vi "ChiSquareCalculation Uncalibrated Method.vi"(9 "refractive index, imaginary":dbl=0.037 format="%.5f", 10 "refractive index, real":dbl=1.567 format="%.5f", 11 "Extinction ExtinctionUncertainity Size parameter and Number ofS sizes 2":T2={"Extinction"=[1.8535327e-09, 2.3370865e-09, 2.8756633e-09, 3.369798e-09, 3.9789465e-09], "Extinction Uncertainty"=[2.1120453e-11, 4.1097261e-11, 5.5818728e-11, 7.3813344e-11, 9.5925372e-11], "Size parameters"=[2.3425015041273096, 2.5554561863207015, 2.7684108685140933, 2.9813655507074848, 3.194320232900877], "Number ofSizes"=5.0, "GeometricCrossSection"=[5.939573610693203e-10, 7.068583470577035e-10, 8.295768100885549e-10, 9.621127501618742e-10, 1.1044661672776617e-09], "Wave Length"=368.81, "SMPS Sizes"=[105.5, 109.4, 113.4, 117.6, 121.9, 126.3, 131.0, 135.8, 140.7, 145.9, 151.2, 156.8, 162.5, 168.5, 174.7, 181.1, 187.7, 194.6, 201.7, 209.1, 216.7, 224.7, 232.9, 241.4, 250.3, 259.5, 269.0, 278.8, 289.0, 299.6, 310.6, 322.0, 333.8, 346.0, 358.7, 371.8, 385.4, 399.5, 414.2, 429.4, 445.1, 461.4, 478.3, 495.8, 514.0, 532.8, 552.3, 572.5, 593.5, 615.3, 637.8, 661.2, 685.4, 710.5, 736.5, 763.5, 791.5], "Concentration"=[[0.0, 0.0, 0.0, 0.0, 0.0, 0.0, 0.0, 0.0, 0.0, 0.0, 0.0, 0.0, 0.0, 0.0, 0.0, 0.0, 0.0, 0.0, 0.0, 0.0, 0.0, 0.0, 0.0, 0.00638904, 0.0448604, 0.138777, 0.238948, 0.258203, 0.179447, 0.0783806, 0.0207428, 0.00279106, 0.000128936, 0.0, 0.0, 0.0, 0.0, 0.00019549, 0.00132468, 0.00397525, 0.00699496, 0.00773861, 0.00587311, 0.00303416, 0.00102868, 0.000183263, 2.21568e-05, 5.32123e-05, 0.000149497, 0.000216876, 0.00023158, 0.000165064, 9.50711e-05, 3.99013e-05, 8.12868e-06, 1.38253e-06, 1.50421e-07], [0.0, 0.0, 0.0, 0.0, 0.0, 0.0, 0.0, 0.0, 0.0, 0.0, 0.0, 0.0, 0.0, 0.0, 0.0, 0.0, 0.0, 0.0, 0.0, 0.0, 0.0, 0.0, 0.0, 0.0, 0.0, 0.00685673, 0.0470895, 0.141594, 0.242879, 0.258016, 0.178865, 0.0777681, 0.0205487, 0.00285525, 0.000153554, 0.0, 0.0, 0.0, 0.0, 0.000111464, 0.00081094, 0.00255922, 0.00482553, 0.00593792, 0.00495016, 0.00247994, 0.000820378, 0.000203601, 2.54423e-05, 1.65921e-05, 5.51241e-05, 0.000106166, 0.000152004, 0.000157397, 8.55848e-05, 5.09931e-05, 2.62187e-05], [0.0, 0.0, 0.0, 0.0, 0.0, 0.0, 0.0, 0.0, 0.0, 0.0, 0.0, 0.0, 0.0, 0.0, 0.0, 0.0, 0.0, 0.0, 0.0, 0.0, 0.0, 0.0, 0.0, 0.0, 0.0, 0.0, 0.0, 0.0072478, 0.0494094, 0.145408, 0.247245, 0.258864, 0.175884, 0.0757159, 0.0204247, 0.00297997, 0.000182238, 0.0, 0.0, 0.0, 0.0, 4.50403e-05, 0.000404956, 0.00155479, 0.00339027, 0.0041382, 0.00335173, 0.00222974, 0.000866046, 0.000189774, 2.77835e-05, 5.5897e-06, 2.322e-05, 6.96631e-05, 9.61216e-05, 0.000135395, 0.000110007], [0.0, 0.0, 0.0, 0.0, 0.0, 0.0, 0.0, 0.0, 0.0, 0.0, 0.0, 0.0, 0.0, 0.0, 0.0, 0.0, 0.0, 0.0, 0.0, 0.0, 0.0, 0.0, 0.0, 0.0, 0.0, 0.0, 0.0, 0.0, 0.0, 0.00780939, 0.0525691, 0.151633, 0.250554, 0.256059, 0.173088, 0.0742833, 0.0201712, 0.00304534, 0.000198007, 0.0, 0.0, 0.0, 0.0, 0.0, 0.000142408, 0.000753018, 0.00176172, 0.00291712, 0.00270485, 0.00146477, 0.000603494, 0.000160512, 3.03021e-05, 5.16487e-06, 8.63352e-06, 1.98837e-05, 1.88692e-05], [0.0, 0.0, 0.0, 0.0, 0.0, 0.0, 0.0, 0.0, 0.0, 0.0, 0.0, 0.0, 0.0, 0.0, 0.0, 0.0, 0.0, 0.0, 0.0, 0.0, 0.0, 0.0, 0.0, 0.0, 0.0, 0.0, 0.0, 0.0, 0.0, 0.0, 0.0, 0.00842444, 0.0550216, 0.154463, 0.252616, 0.255039, 0.17071, 0.0735065, 0.0199664, 0.0030828, 0.00020951, 0.0, 0.0, 0.0, 0.0, 0.0, 7.86166e-05, 0.000514629, 0.00130646, 0.001695, 0.00160924, 0.00101698, 0.000516856, 0.000187962, 3.12302e-05, 3.4942e-06, 0.0]], "Double Charge Correction"=TRUE, "Extincation Factor"=1.0, "Diameter Factor"=1.0, "Diameter Offset"=0.0, "Extinction Factor Flag"=FALSE, "Diameter Factor Flag"=FALSE, "Diameter Offset Flag"=FALSE, "Sizes"=[275.0, 300.0, 325.0, 350.0, 375.0], "ExtinctionOrAbsorptionOrScattering"=0, "Concentration(#/cc)"=[]} {"ExtinctionOrAbsorptionOrScattering" scale=0.0..2.0}) -> (1 "slope of Uncalibrated Data":dbl, 2 "Predicted Absorption Coef":dbl[](array[numeric]), 3 "Chi Squared":dbl=0.43514880104819414)   [LabVIEW 2013]
uses:
  BaesDataTypeDefinition.ctl
  <vilib>/Analysis/6fits.llb/Curve Fitting Criteria.ctl
  <vilib>/Analysis/NI_AALPro.lvlib
panel:
  out "Extinction Graph":T1(graph)=[{"Ramp Pattern"=[2.3425015041273096, 2.5554561863207015, 2.7684108685140933, 2.9813655507074848, 3.194320232900877], "Extinction"=[1.8535327e-09, 2.3370865e-09, 2.8756633e-09, 3.369798e-09, 3.9789465e-09]}, {"Ramp Pattern"=[2.3425015041273096, 2.5554561863207015, 2.7684108685140933, 2.9813655507074848, 3.194320232900877], "Extinction"=[1.8559851433508356e-09, 2.3367650037187104e-09, 2.8534894447318493e-09, 3.3654949938011214e-09, 4.027896682856635e-09]}]
  # "Output"
  # "Mie scattering demo program, August 2005, by Martin Fierz (martin@fierz.ch)\n\nThis VI demonstrates the usage of mie2.dll; a dynamic-link-library which you can call in your LabView program.\nThe demo lets you select the refractive index of a sphere, and the size parameter and computes total scattering,\ntotal extinction and angular distribution of the scattered light for p-, s- and unpolarized light.\nMie2.dll uses the Bohren-Huffman Mie code."
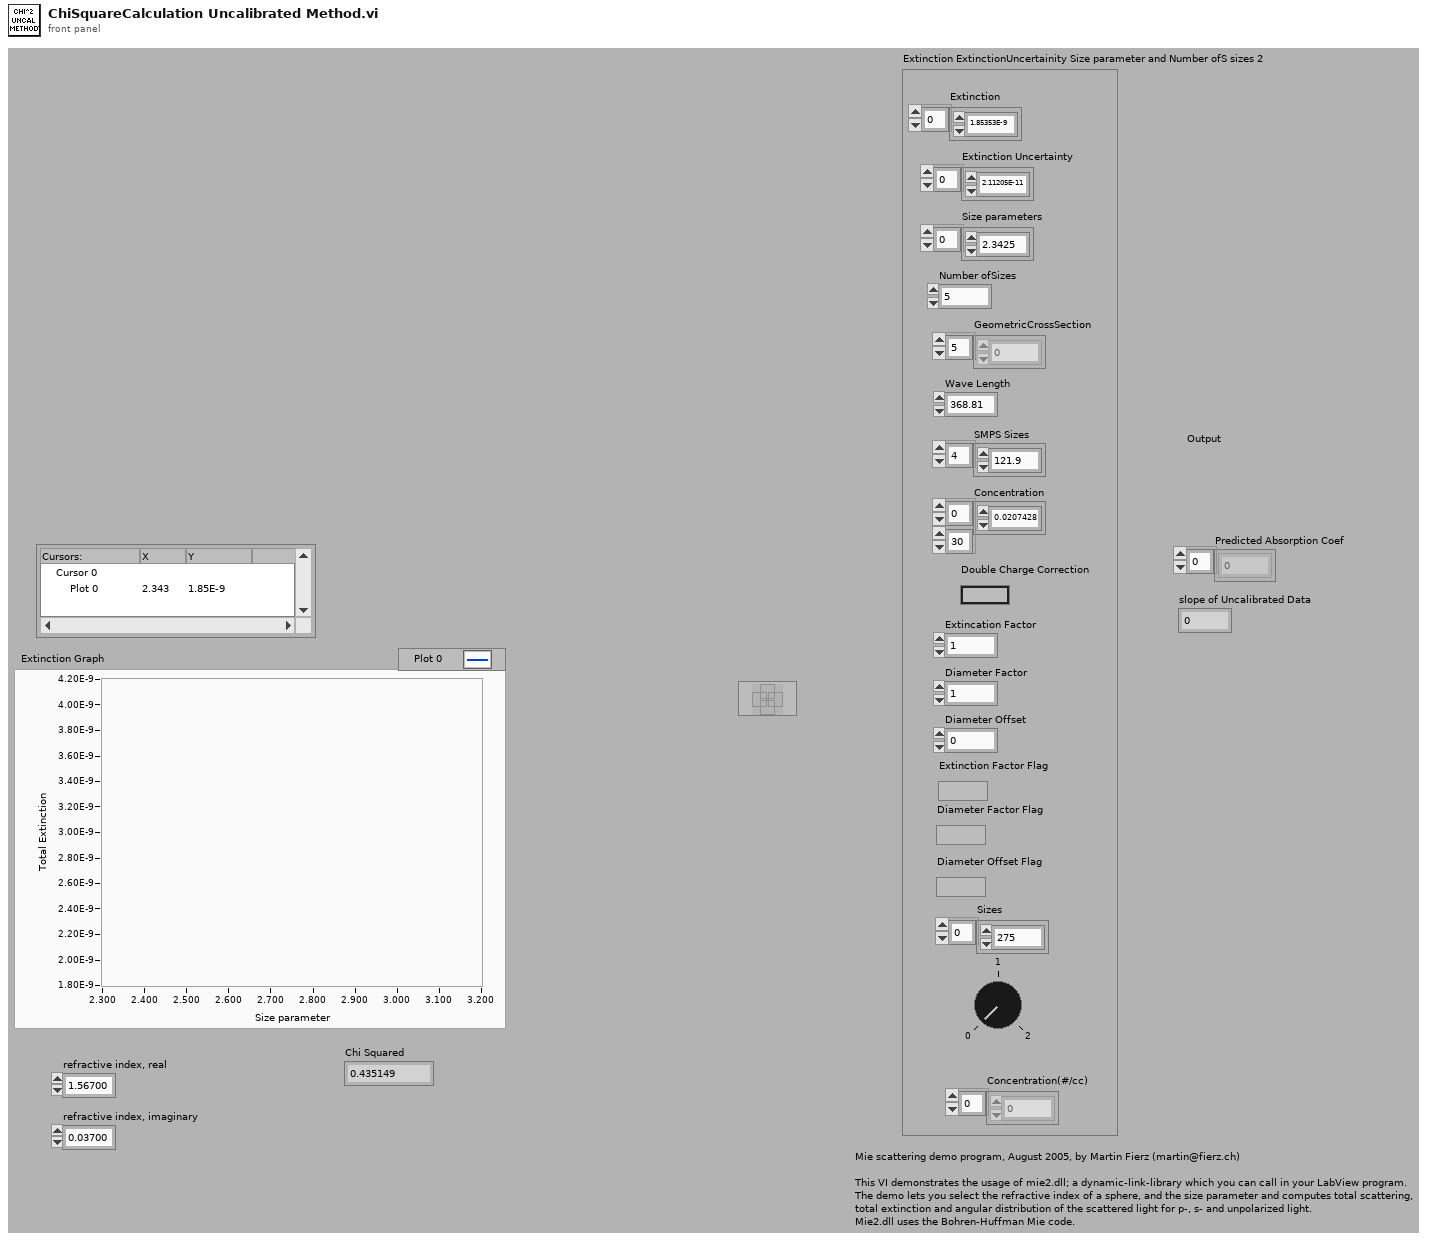
[diagram p1: front panel]
types:
  T1 = cluster{"Ramp Pattern":dbl[], "Extinction":dbl[]}[]
  T2 = typedef "BaesDataTypeDefinition.ctl" = cluster{"Extinction":dbl[], "Extinction Uncertainty":dbl[], "Size parameters":dbl[], "Number ofSizes":dbl, "GeometricCrossSection":dbl[], "Wave Length":dbl, "SMPS Sizes":dbl[], "Concentration":dbl[][], "Double Charge Correction":bool, "Extincation Factor":dbl, "Diameter Factor":dbl, "Diameter Offset":dbl, "Extinction Factor Flag":bool, "Diameter Factor Flag":bool, "Diameter Offset Flag":bool, "Sizes":dbl[], "ExtinctionOrAbsorptionOrScattering":i8, "Concentration(#/cc)":dbl[]}
  T3 = typedef "NI_AALPro.lvlib/Curve Fitting Criteria.ctl" = u16
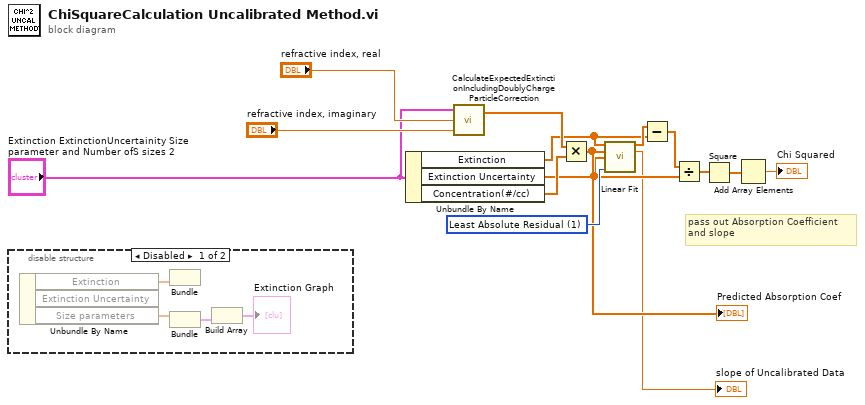
[diagram p0: block diagram]
diagram:
  w11 = T3 1 items=["Least Square", "Least Absolute Residual", "Bisquare"] ("method")
  # "pass out Absorption Coefficient\nand slope"
  n1 = disable-structure shown="Disabled" {
    frame Disabled {
      n2 = Unbundle By Name() -> ("Extinction"=w16:dbl[], "Size parameters"=w18:dbl[])  [unwired: 1 in, 1 out]
      n3 = Bundle("Extinction"=w16) -> ()  [unwired: 2 in, 1 out]
      n4 = Bundle("Size parameters"=w18) -> (w19:cluster{"Size parameters":dbl[], void})  [unwired: 2 in]
      n5 = Build Array(w19) -> (→"Extinction Graph":cluster{"Size parameters":dbl[], void}[], w17:cluster{"Size parameters":dbl[], void})
    }
    frame Enabled {
    }
  }
  n6 = Unbundle By Name("Extinction ExtinctionUncertainity Size parameter and Number ofS sizes 2") -> ("Extinction"=w8:dbl[], "Extinction Uncertainty"=w4:dbl[], "Concentration(#/cc)"=w12:dbl[])
  n7 = call "CalculateExpectedExtinctionIncludingDoublyChargeParticleCorrection.vi"("refractive index, imaginary"="refractive index, imaginary", "refractive index, real"="refractive index, real", "Extinction ExtinctionUncertainity Size parameter and Number ofS sizes"="Extinction ExtinctionUncertainity Size parameter and Number ofS sizes 2") -> ("Expected Extinction Cross Section"=w13:sgl[])  [unwired: 1 out]
  n8 = Multiply(x=w13, y=w12) -> (x*y=w10:dbl[])
  "Predicted Absorption Coef" <- w10
  n9 = call <vilib>:"Linear Fit.vi"("Y"=w8, "X"=w10, "Weight"=w4, "method"=w11) -> ("Best Linear Fit"=w9:dbl[], "slope"=→"slope of Uncalibrated Data":dbl)  [unwired: 7 in, 3 out]
  n10 = Subtract(x=w9, y=w8) -> (x-y=w7:dbl[])
  n11 = Divide(x=w7, y=w4) -> (x/y=w6:dbl[])
  n12 = Square(x=w6) -> (x^2=w5:dbl[])
  n13 = Add Array Elements(numeric array=w5) -> (sum=→"Chi Squared":dbl)
